vi "Uploading Multiple Audio Files to ELVIS.vi"() -> ()   [LabVIEW 2019]
doc: "This VI converts all the music files inside a folder to a readable NI ELVIS III files. After making the convertion, each file is saved into the projects folder and then transfered to the target."
uses:
  Uploading to ELVIS Global Variables.vi
panel:
  in  "Stop":bool
  out "Current File":string
  out "error out":errorcluster
  out "Signal Out":dbl(graph) caption="Audio Signal Out"
  out "Status":string
  in  "error in (no error)":errorcluster
  in  "Host ID":string="172.22.11.2"
  in  "Music Files Folder":path=path "C:/Users/NI 2019/Desktop/Audio Modulation and Demodulation/Audio"
  # "Creating and Uploading multiple audio files into a NI ELVIS III"
  # "This VI converts all the music files inside a folder to a readable NI ELVIS III files. After making the convertion, each file is saved into the projects folder and then transfered to the target.\n\nRemember to use this VI for transfering the music or audio files before running any of the Audio VIs on the equipment.\n\nThe data tranference might take a while. Please, do not abort the VI or disconnect the target while this VI is running. The Stop button only works after finalizing transfering the song."
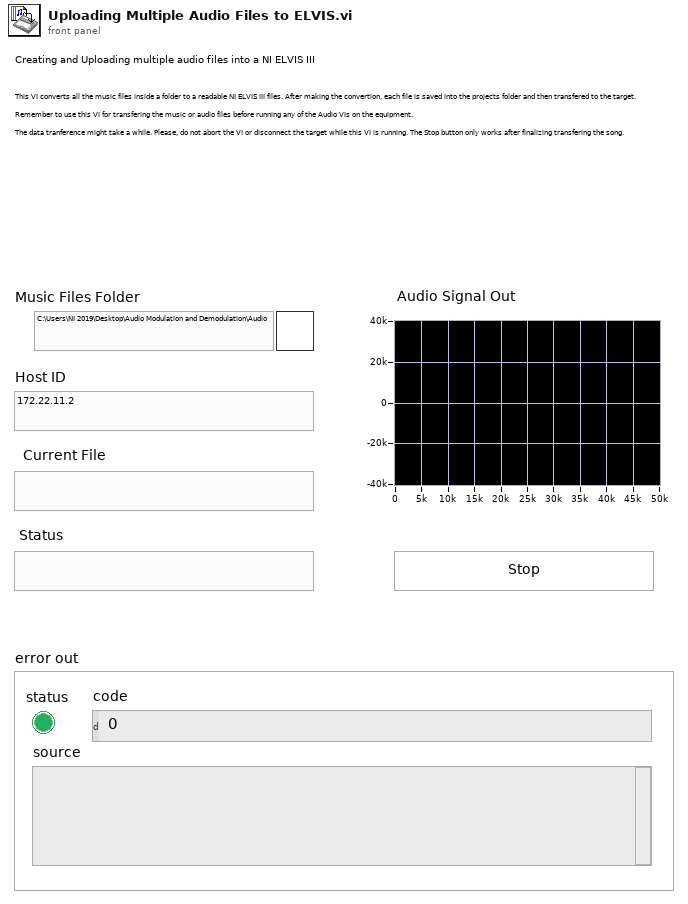
[diagram p1: front panel]
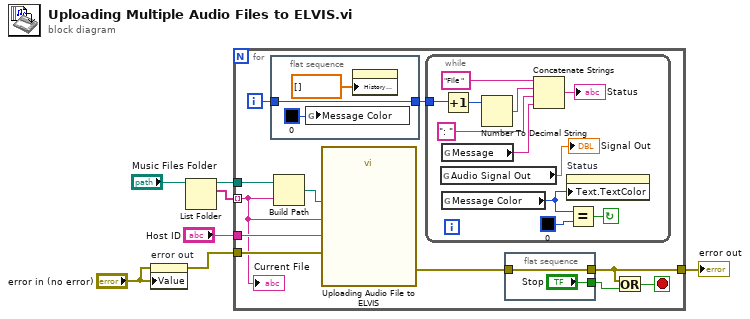
[diagram p0: block diagram]
diagram:
  n1 = property on="error out" class="Clust (strict)"(error in="error in (no error)", "Value"="error in (no error)") -> (error out=w2:errorcluster)  [unwired: 1 in, 1 out]
  n2 = List Folder(path="Music Files Folder") -> (path out=w4:path, filenames=w6:string[])  [unwired: 3 in, 2 out]
  n3 = for {
    tunnel: w6 -> [w12] mode=indexing
    tunnel: "Host ID" -> [w18]
    tunnel: w4 -> [w17]
    tunnel: w2 -> [w15]
    tunnel: [w8] -> w3
    i -> [w14]
    stop <- w9 stop-if-true
    n4 = flat-sequence {
      tunnel: w14 -> [w22]
      tunnel: [w22] -> w13
      frame #0 {
        n5 = global write "Uploading to ELVIS Global Variables.vi" "Message Color"(u32 0 ("Text.Text Colors:Text Color")) -> ()
        n6 = property on="Signal Out" class="WFChart (strict)"("History Data"=dbl[] []) -> ()  [unwired: 2 in, 2 out]
      }
    }
    n7 = Build Path(base path=w17, name or relative path=w12) -> (appended path=w16:path)
    n8 = call "Uploading Audio File to ELVIS.vi"("error in (no error)"=w15, "Host ID"=w18, "New File Name"=w12, "Music File"=w16) -> ("error out"=w11:errorcluster)  [unwired: 7 in]
    n9 = while {
      tunnel: w13 -> [w24]
      stop <- w33 continue-if-true
      n10 = global read "Uploading to ELVIS Global Variables.vi" "Audio Signal Out"() -> (→"Signal Out":dbl)
      n11 = global read "Uploading to ELVIS Global Variables.vi" "Message"() -> (w29:string)
      n12 = global read "Uploading to ELVIS Global Variables.vi" "Message Color"() -> (w27:u32)
      n13 = Increment(x=w24) -> (x+1=w26:i32)
      n14 = Number To Decimal String(number=w26) -> (decimal integer string=w31:string)  [unwired: 1 in]
      n15 = Concatenate Strings("File ", w31, ": ", w29) -> (→"Status":string)
      n16 = property on="Status" class="Str"("Text.TextColor"=w27) -> ()  [unwired: 2 in, 2 out]
      n17 = Equal?(x=w27, y=u32 0 ("Text.Text Colors:Text Color")) -> (x = y?=w33:bool)
    }
    n18 = flat-sequence {
      tunnel: ["Stop"] -> w10
      tunnel: [w19] -> w8
      tunnel: w11 -> [w19]
      frame #0 {
      }
    }
    n19 = Or(x=w8, y=w10) -> (x .or. y?=w9:bool)
    "Current File" <- w12
  }
  "error out" <- w3
